vi "Init - Add DataReplayLoops.vi"(8 "error in (no error)":errorcluster, 10 "DataReplay Components":T1[](array[typedef]), 11 "Crank Cams Page in":T3 format="%.0x") -> (0 "error out":errorcluster, 3 "Crank Cams Page out":T3 format="%.0x")   [LabVIEW 2011, in "Engine Sim System Explorer.lvlib"]
uses:
  Engine Sim System Explorer.lvlib
  <vilib>/NI Veristand/Custom Device API/Custom Device Item Ref.ctl
  TypeDefs/DataReplayLoopComp.ctl
  TypeDefs/DataReplayComp.ctl
  Add Data Replay.vi
  Shared/Engine Simulation Global.vi
  <vilib>/NI Veristand/Custom Device API/NI VeriStand - Add Custom Device Section.vi
  <vilib>/NI Veristand/Custom Device API/NI VeriStand - Add Custom Device Channel.vi
  <vilib>/NI Veristand/Custom Device API/Custom Device API.lvlib
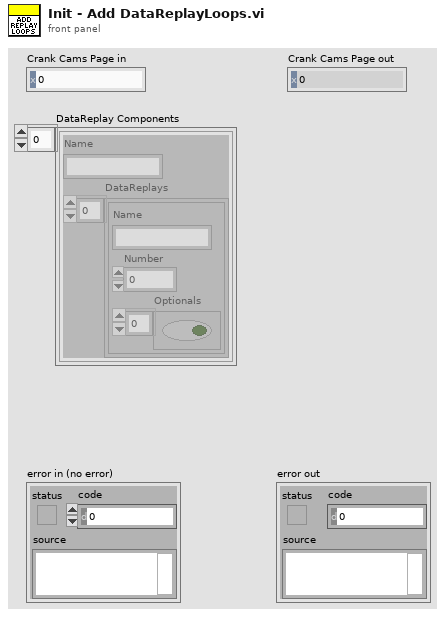
[diagram p1: front panel]
types:
  T1 = typedef "Engine Sim System Explorer.lvlib/DataReplayLoopComp.ctl" = cluster{"Name":string, "DataReplays":T2[]}
  T2 = typedef "Engine Sim System Explorer.lvlib/DataReplayComp.ctl" = cluster{"Name":string, "Number":i8, "Optionals":bool[]}
  T3 = typedef "Custom Device API.lvlib/Custom Device Item Ref.ctl" = u64
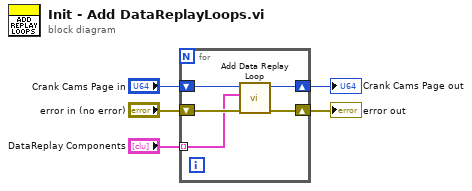
[diagram p0: block diagram]
diagram:
  n1 = for {
    shift-right: [w6] -> w1
    shift-left: "Crank Cams Page in" -> [w10]
    shift-right: [w7] -> w2
    shift-left: "error in (no error)" -> [w9]
    tunnel: "DataReplay Components" -> [w8] mode=indexing
    n2 = call "Add Data Replay Loop.vi"("error in (no error)"=w9, "DataReplay Loop"=w8, "Crank Cams Page in"=w10) -> ("error out"=w7:errorcluster, "Parent Ref out"=w6:T3)  [unwired: 7 in]
  }
  "error out" <- w2
  "Crank Cams Page out" <- w1
